vi "pmu_Compute Reported Phasors.vi"(8 "error in (no error)":errorcluster, 9 "PMU system info in":refnum<class "PMU System Info.lvclass">, 11 "physical channel phasors":csg[](array[numeric])) -> (0 "error out":errorcluster, 1 "PMU system info out":refnum<class "PMU System Info.lvclass">, 3 "reported phasors":csg[](array[numeric]))   [LabVIEW 2014, in "NI_EP_PMU.lvlib"]
uses:
  <vilib>/addons/Electrical Power/PMU/NI_EP_PMU.lvlib
  <vilib>/addons/Electrical Power/PMU/Common/Classes/PMU System Info/PMU System Info.lvclass
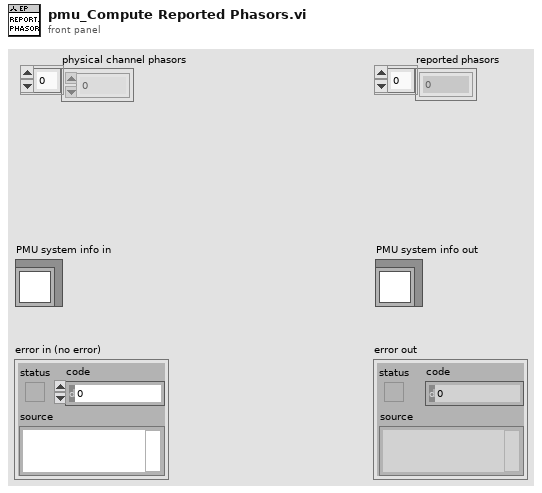
[diagram p1: front panel]
types:
  T1 = typedef "NI_EP_PMU.lvlib/pmu_Phasor Channel Info.ctl" = cluster{"channel indexes":i32[], "phasor phase":enum16{"Phase A (L1)", "Phase B (L2)", "Phase C (L3)", "Phase N", "Positive sequence", "Negative sequence", "Zero sequence"}, "connection type":enum16{"Wye", "Delta"}}
  T2 = enum16{"Phase A (L1)", "Phase B (L2)", "Phase C (L3)", "Phase N", "Positive sequence", "Negative sequence", "Zero sequence"}
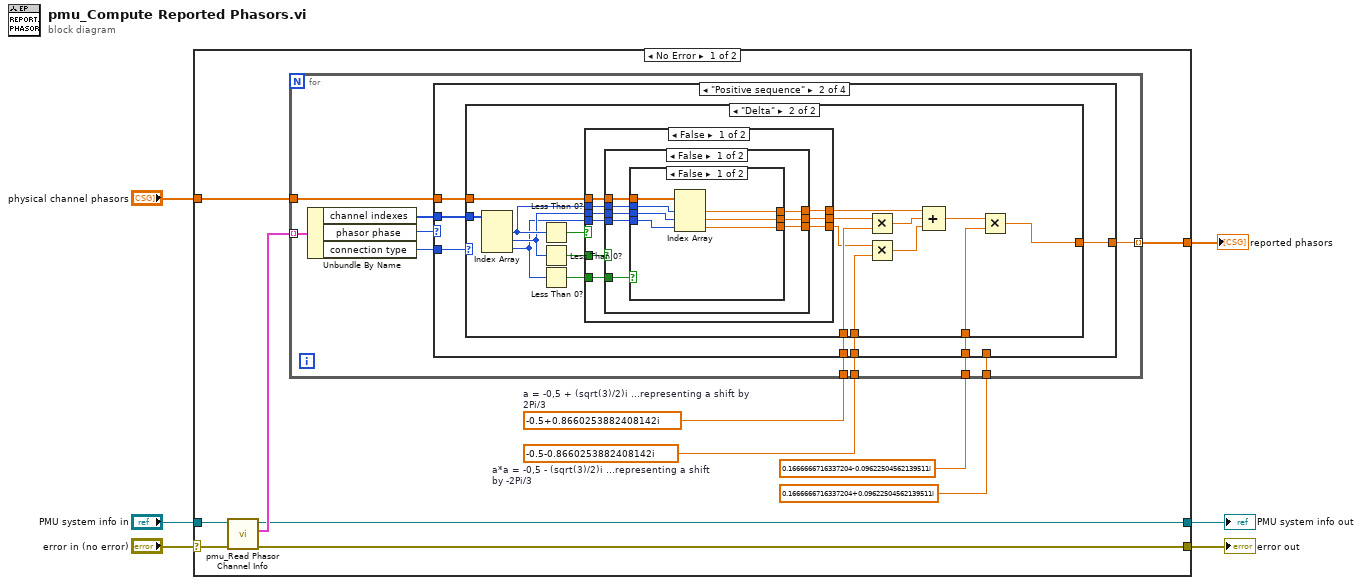
[diagram p0: block diagram]
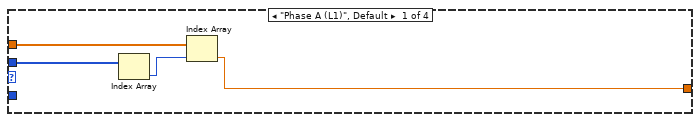
[diagram p2: hidden frame]
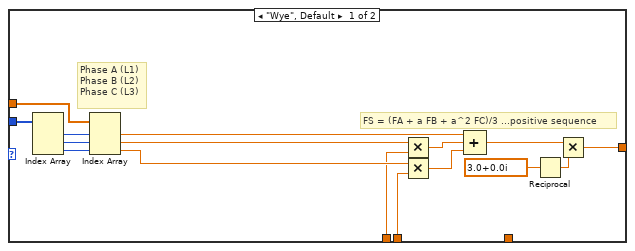
[diagram p3: hidden frame]
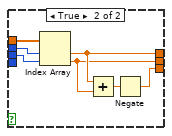
[diagram p4: hidden frame]
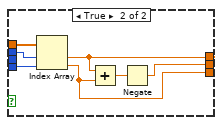
[diagram p5: hidden frame]
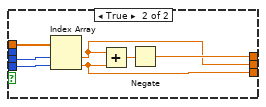
[diagram p6: hidden frame]
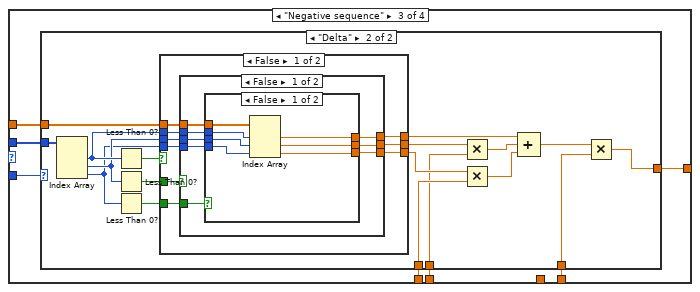
[diagram p7: hidden frame]
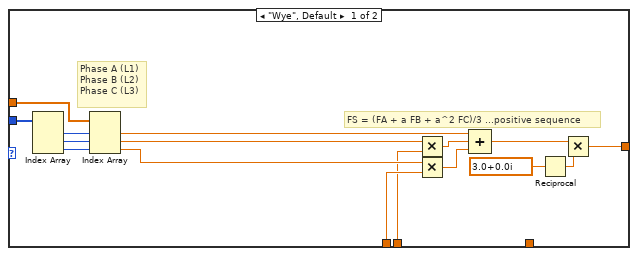
[diagram p8: hidden frame]
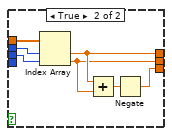
[diagram p9: hidden frame]
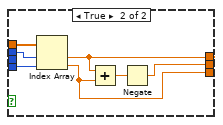
[diagram p10: hidden frame]
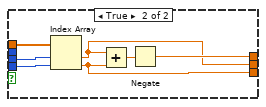
[diagram p11: hidden frame]
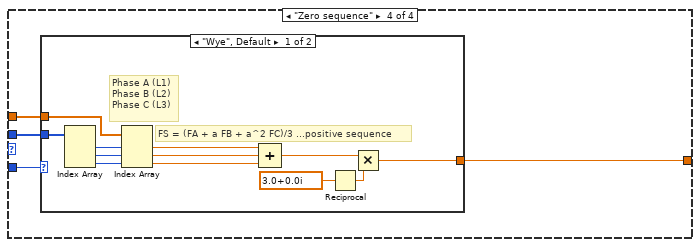
[diagram p12: hidden frame]
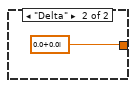
[diagram p13: hidden frame]
diagram:
  n1 = case shown="No Error" "error in (no error)" {
    selector: "error in (no error)" -> [w13 w222]
    tunnel: "physical channel phasors" -> [w17 _]
    tunnel: [w16 _] -> w1
    tunnel: [w12 w222] -> w2
    tunnel: "PMU system info in" -> [w14 w221]
    tunnel: [w11 w221] -> w3
    frame No Error {
      w9 = csg -0.5-0.8660254i  # a*a = -0,5 - (sqrt(3)/2)i ...representing a shift by -2Pi/3
      w10 = csg -0.5+0.8660254i  # a = -0,5 + (sqrt(3)/2)i ...representing a shift by 2Pi/3
      n2 = call <vilib>:"pmu_Read Phasor Channel Info.vi"("error in (no error)"=w13, "system info in"=w14) -> ("error out"=w12:errorcluster, "phasor channel info"=w15:T1[], "system info out"=w11:refnum<class "PMU System Info.lvclass">)  [unwired: 7 in]
      n3 = for {
        tunnel: w17 -> [w27]
        tunnel: [w26] -> w16 mode=indexing
        tunnel: w15 -> [w25] mode=indexing
        tunnel: w10 -> [w22]
        tunnel: w9 -> [w21]
        tunnel: csg 0.16666667-0.096225046i -> [w19]
        tunnel: csg 0.16666667+0.096225046i -> [w18]
        n4 = Unbundle By Name(w25) -> ("channel indexes"=w24:i32[], "phasor phase"=w23:T2, "connection type"=w20:enum16{"Wye", "Delta"})
        n5 = case shown="\"Positive sequence\"" w23 {
          tunnel: w27 -> [w31 w35 w121 w206]
          tunnel: [w30 w38 w124 w207] -> w26
          tunnel: w22 -> [_ w37 w123 _]
          tunnel: w21 -> [_ w36 w122 _]
          tunnel: w24 -> [w29 w34 w120 w205]
          tunnel: w20 -> [_ w33 w119 w204]
          tunnel: w19 -> [_ w32 _ _]
          tunnel: w18 -> [_ _ w118 _]
          frame "Phase A (L1)", Default {
            n6 = Index Array(array=w29) -> (element=w28:i32)  [unwired: 1 in]
            n7 = Index Array(array=w31, index=w28) -> (element=w30:csg)
          }
          frame "Positive sequence" {
            n8 = case shown="\"Delta\"" w33 {
              tunnel: [w46 w55] -> w38
              tunnel: w37 -> [w45 w63]
              tunnel: w36 -> [w44 w61]
              tunnel: w35 -> [w43 w68]
              tunnel: w34 -> [w42 w72]
              tunnel: w32 -> [_ w56]
              frame "Wye", Default {
                # "FS = (FA + a FB + a^2 FC)/3 ...positive sequence"
                # "Phase A (L1)\nPhase B (L2)\nPhase C (L3)"
                n9 = Index Array(array=w42) -> (element #1=w41:i32, element #2=w40:i32, element #3=w39:i32)  [unwired: 3 in]
                n10 = Index Array(array=w43, index #1=w41, index #2=w40, index #3=w39) -> (element #1=w47:csg, element #2=w51:csg, element #3=w50:csg)
                n11 = Multiply(x=w51, y=w45) -> (x*y=w49:csg)
                n12 = Multiply(x=w50, y=w44) -> (x*y=w48:csg)
                n13 = Compound Arithmetic op=ADD(w47, w49, w48) -> (w53:csg)
                n14 = Reciprocal(x=csg 3.0+0.0i ("y")) -> (1/x=w52:csg)
                n15 = Multiply(x=w53, y=w52) -> (x*y=w46:csg)
              }
              frame "Delta" {
                n16 = Index Array(array=w72) -> (element #1=w67:i32, element #2=w66:i32, element #3=w65:i32)  [unwired: 3 in]
                n17 = Less Than 0?(x=w67) -> (x < 0?=w71:bool)
                n18 = Less Than 0?(x=w66) -> (x < 0?=w70:bool)
                n19 = Less Than 0?(x=w65) -> (x < 0?=w69:bool)
                n20 = case shown="False" w71 {
                  tunnel: w70 -> [w81 _]
                  tunnel: w69 -> [w77 _]
                  tunnel: w68 -> [w80 w117]
                  tunnel: w67 -> [w79 _]
                  tunnel: w66 -> [w76 w116]
                  tunnel: w65 -> [w78 w115]
                  tunnel: [w75 w113] -> w60
                  tunnel: [w74 w112] -> w64
                  tunnel: [w73 w111] -> w62
                  frame False {
                    n21 = case shown="False" w81 {
                      tunnel: w80 -> [w88 w110]
                      tunnel: w79 -> [w87 w109]
                      tunnel: w78 -> [w85 w108]
                      tunnel: w77 -> [w89 _]
                      tunnel: w76 -> [w86 _]
                      tunnel: [w84 w106] -> w75
                      tunnel: [w83 w105] -> w74
                      tunnel: [w82 w104] -> w73
                      frame False {
                        n22 = case shown="False" w89 {
                          tunnel: w88 -> [w96 w103]
                          tunnel: w87 -> [w95 w102]
                          tunnel: w86 -> [w94 w101]
                          tunnel: w85 -> [w93 _]
                          tunnel: [w92 w99] -> w84
                          tunnel: [w91 w98] -> w83
                          tunnel: [w90 w97] -> w82
                          frame False {
                            n23 = Index Array(array=w96, index #1=w95, index #2=w94, index #3=w93) -> (element #1=w92:csg, element #2=w91:csg, element #3=w90:csg)
                          }
                          frame True {
                            n24 = Index Array(array=w103, index #1=w102, index #2=w101) -> (element #1=w99:csg, element #2=w98:csg)
                            n25 = Add(x=w99, y=w98) -> (x+y=w100:csg)
                            n26 = Negate(x=w100) -> (-x=w97:csg)
                          }
                        }
                      }
                      frame True {
                        n27 = Index Array(array=w110, index #1=w109, index #2=w108) -> (element #1=w106:csg, element #2=w104:csg)
                        n28 = Add(x=w106, y=w104) -> (x+y=w107:csg)
                        n29 = Negate(x=w107) -> (-x=w105:csg)
                      }
                    }
                  }
                  frame True {
                    n30 = Index Array(array=w117, index #1=w116, index #2=w115) -> (element #1=w112:csg, element #2=w111:csg)
                    n31 = Add(x=w112, y=w111) -> (x+y=w114:csg)
                    n32 = Negate(x=w114) -> (-x=w113:csg)
                  }
                }
                n33 = Multiply(x=w64, y=w63) -> (x*y=w59:csg)
                n34 = Multiply(x=w62, y=w61) -> (x*y=w58:csg)
                n35 = Compound Arithmetic op=ADD(w60, w59, w58) -> (w57:csg)
                n36 = Multiply(x=w57, y=w56) -> (x*y=w55:csg)
              }
            }
          }
          frame "Negative sequence" {
            n37 = case shown="\"Delta\"" w119 {
              tunnel: [w132 w144] -> w124
              tunnel: w123 -> [w126 w143]
              tunnel: w122 -> [w125 w142]
              tunnel: w121 -> [w131 w154]
              tunnel: w120 -> [w130 w158]
              tunnel: w118 -> [_ w141]
              frame "Wye", Default {
                # "FS = (FA + a FB + a^2 FC)/3 ...positive sequence"
                # "Phase A (L1)\nPhase B (L2)\nPhase C (L3)"
                n38 = Index Array(array=w130) -> (element #1=w129:i32, element #2=w128:i32, element #3=w127:i32)  [unwired: 3 in]
                n39 = Index Array(array=w131, index #1=w129, index #2=w128, index #3=w127) -> (element #1=w133:csg, element #2=w137:csg, element #3=w136:csg)
                n40 = Multiply(x=w137, y=w125) -> (x*y=w135:csg)
                n41 = Multiply(x=w136, y=w126) -> (x*y=w134:csg)
                n42 = Compound Arithmetic op=ADD(w133, w135, w134) -> (w139:csg)
                n43 = Reciprocal(x=csg 3.0+0.0i ("y")) -> (1/x=w138:csg)
                n44 = Multiply(x=w139, y=w138) -> (x*y=w132:csg)
              }
              frame "Delta" {
                n45 = Index Array(array=w158) -> (element #1=w153:i32, element #2=w152:i32, element #3=w151:i32)  [unwired: 3 in]
                n46 = Less Than 0?(x=w153) -> (x < 0?=w157:bool)
                n47 = Less Than 0?(x=w152) -> (x < 0?=w156:bool)
                n48 = Less Than 0?(x=w151) -> (x < 0?=w155:bool)
                n49 = case shown="False" w157 {
                  tunnel: w156 -> [w167 _]
                  tunnel: w155 -> [w163 _]
                  tunnel: w154 -> [w166 w203]
                  tunnel: w153 -> [w165 _]
                  tunnel: w152 -> [w162 w202]
                  tunnel: w151 -> [w164 w201]
                  tunnel: [w161 w199] -> w148
                  tunnel: [w160 w198] -> w150
                  tunnel: [w159 w197] -> w149
                  frame False {
                    n50 = case shown="False" w167 {
                      tunnel: w166 -> [w174 w196]
                      tunnel: w165 -> [w173 w195]
                      tunnel: w164 -> [w171 w194]
                      tunnel: w163 -> [w175 _]
                      tunnel: w162 -> [w172 _]
                      tunnel: [w170 w192] -> w161
                      tunnel: [w169 w191] -> w160
                      tunnel: [w168 w190] -> w159
                      frame False {
                        n51 = case shown="False" w175 {
                          tunnel: w174 -> [w182 w189]
                          tunnel: w173 -> [w181 w188]
                          tunnel: w172 -> [w180 w187]
                          tunnel: w171 -> [w179 _]
                          tunnel: [w178 w185] -> w170
                          tunnel: [w177 w184] -> w169
                          tunnel: [w176 w183] -> w168
                          frame False {
                            n52 = Index Array(array=w182, index #1=w181, index #2=w180, index #3=w179) -> (element #1=w178:csg, element #2=w177:csg, element #3=w176:csg)
                          }
                          frame True {
                            n53 = Index Array(array=w189, index #1=w188, index #2=w187) -> (element #1=w185:csg, element #2=w184:csg)
                            n54 = Add(x=w185, y=w184) -> (x+y=w186:csg)
                            n55 = Negate(x=w186) -> (-x=w183:csg)
                          }
                        }
                      }
                      frame True {
                        n56 = Index Array(array=w196, index #1=w195, index #2=w194) -> (element #1=w192:csg, element #2=w190:csg)
                        n57 = Add(x=w192, y=w190) -> (x+y=w193:csg)
                        n58 = Negate(x=w193) -> (-x=w191:csg)
                      }
                    }
                  }
                  frame True {
                    n59 = Index Array(array=w203, index #1=w202, index #2=w201) -> (element #1=w198:csg, element #2=w197:csg)
                    n60 = Add(x=w198, y=w197) -> (x+y=w200:csg)
                    n61 = Negate(x=w200) -> (-x=w199:csg)
                  }
                }
                n62 = Multiply(x=w150, y=w142) -> (x*y=w147:csg)
                n63 = Multiply(x=w149, y=w143) -> (x*y=w146:csg)
                n64 = Compound Arithmetic op=ADD(w148, w147, w146) -> (w145:csg)
                n65 = Multiply(x=w145, y=w141) -> (x*y=w144:csg)
              }
            }
          }
          frame "Zero sequence" {
            n66 = case shown="\"Wye\", Default" w204 {
              tunnel: [w215 csg 0.0+0.0i] -> w207
              tunnel: w206 -> [w214 _]
              tunnel: w205 -> [w213 _]
              frame "Wye", Default {
                # "FS = (FA + a FB + a^2 FC)/3 ...positive sequence"
                # "Phase A (L1)\nPhase B (L2)\nPhase C (L3)"
                n67 = Index Array(array=w213) -> (element #1=w212:i32, element #2=w211:i32, element #3=w210:i32)  [unwired: 3 in]
                n68 = Index Array(array=w214, index #1=w212, index #2=w211, index #3=w210) -> (element #1=w216:csg, element #2=w209:csg, element #3=w208:csg)
                n69 = Compound Arithmetic op=ADD(w216, w209, w208) -> (w218:csg)
                n70 = Reciprocal(x=csg 3.0+0.0i ("y")) -> (1/x=w217:csg)
                n71 = Multiply(x=w218, y=w217) -> (x*y=w215:csg)
              }
              frame "Delta" {
              }
            }
          }
        }
      }
    }
    frame Error {
    }
  }
  "reported phasors" <- w1
  "error out" <- w2
  "PMU system info out" <- w3
